vi "Thorlabs_CCS_Connection_manager.vi"(0 "Parameter":variant, 2 "Action":T2=enum."Disconnect", 11 "error in":errorcluster) -> (4 "Instrument Refnum":refnum<visa-resource-name>, 6 "Not Connected":bool, 8 "Detector Info":T1, 15 "error out":errorcluster)   [LabVIEW 2021]
doc: "A functional global VI to manage the connection with the instrument"
uses:
  _Controls/Thorlabs_CCS_Connection_manager_action.ctl
  _Controls/Thorlabs_CCS_Detector_Info.ctl
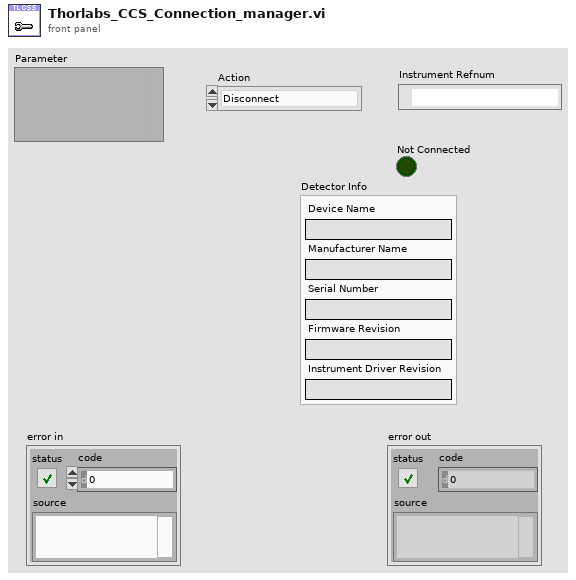
[diagram p1: front panel]
types:
  T1 = typedef "Thorlabs_CCS_Detector_Info.ctl" = cluster{"Device Name":string, "Manufacturer Name":string, "Serial Number":string, "Firmware Revision":string, "Instrument Driver Revision":string}
  T2 = typedef "Thorlabs_CCS_Connection_manager_action.ctl" = enum16{"Get Reference", "Connect", "Disconnect", "Set USB VISA Resource Name "}
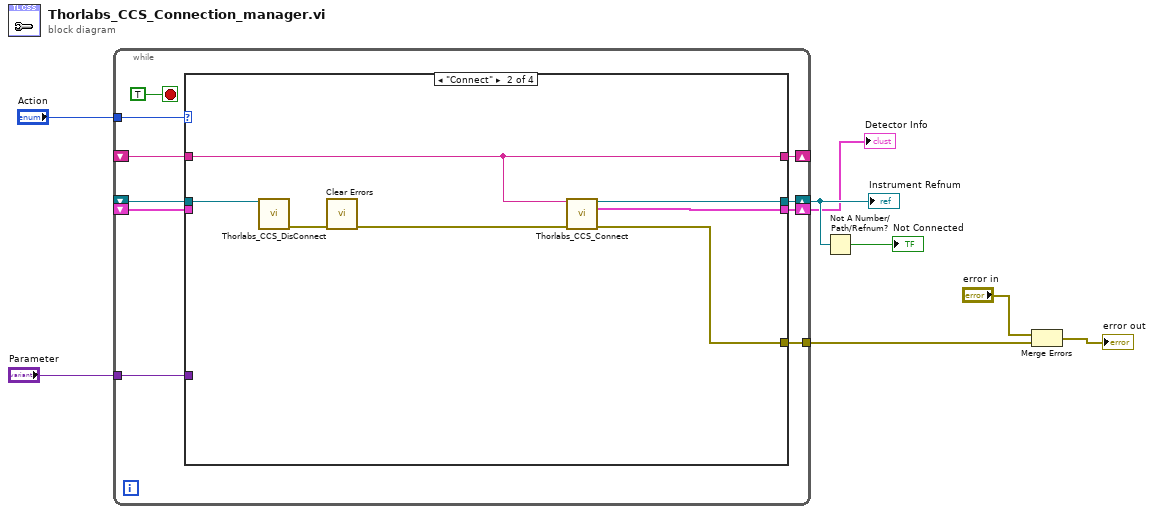
[diagram p0: block diagram]
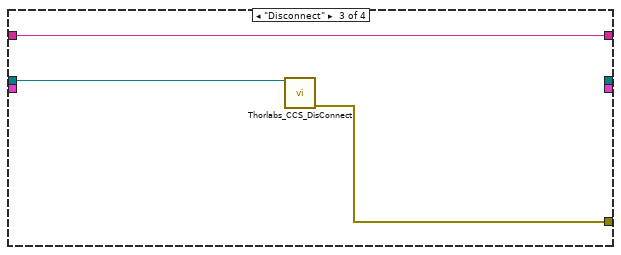
[diagram p3: hidden frame]
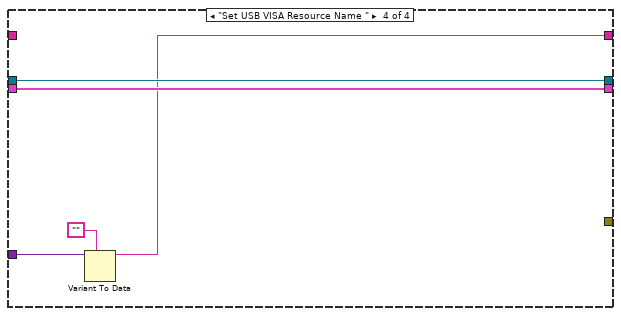
[diagram p4: hidden frame]
diagram:
  n1 = while {
    tunnel: "Action" -> [w17]
    shift-right: [w16] -> w4
    shift-left: _ -> [w15]
    tunnel: [w14] -> w5
    shift-right: [w13] -> w2
    shift-left: _ -> [w12]
    tunnel: "Parameter" -> [w11]
    shift-right: [w10] -> _
    shift-left: _ -> [w9]
    stop <- TRUE stop-if-true
    n2 = case shown="\"Connect\"" w17 {
      tunnel: [w21 w28 _ w35] -> w16
      tunnel: w15 -> [w21 w25 w31 w35]
      tunnel: [_ w27 w30 _] -> w14
      tunnel: [w20 w24 _ w36] -> w13
      tunnel: w12 -> [w20 _ _ w36]
      tunnel: w11 -> [_ _ _ w33]
      tunnel: [w19 w22 w29 w32] -> w10
      tunnel: w9 -> [w19 w22 w29 _]
      frame "Get Reference" {
      }
      frame "Connect" {
        n3 = call "Thorlabs_CCS_DisConnect.vi"("VISA Refnum in"=w25) -> ("error out"=w26:errorcluster)  [unwired: 14 in]
        n4 = call <vilib>:"Clear Errors.vi"("error in (no error)"=w26) -> ("error out"=w23:errorcluster)  [unwired: 5 in, 1 out]
        n5 = call "Thorlabs_CCS_Connect.vi"("USB VISA Resource Name"=w22, "error in (no error)"=w23) -> ("Instrument Refnum"=w28:refnum<visa-resource-name>, "Detector"=w24:T1, "error out"=w27:errorcluster)  [unwired: 11 in]
      }
      frame "Disconnect" {
        n6 = call "Thorlabs_CCS_DisConnect.vi"("VISA Refnum in"=w31) -> ("error out"=w30:errorcluster)  [unwired: 14 in]
      }
      frame "Set USB VISA Resource Name " {
        n7 = Variant To Data(type="", Variant=w33) -> (data=w32:string)  [unwired: 1 in, 1 out]
      }
    }
  }
  "Instrument Refnum" <- w4
  "Detector Info" <- w2
  n8 = Not A Number/Path/Refnum?(number/path/refnum=w4) -> (NaN/Path/Refnum?=→"Not Connected":bool)
  n9 = Merge Errors("error in", w5) -> (→"error out":errorcluster)
